vi "PTSequencer.check stop conditions.vi"(1 "conditions":T1[](array[typedef])) -> (0 "fulfilled":bool)   [LabVIEW 2014, in "PTSequencer.lvlib"]
uses:
  PTSequencer.lvlib
  PTSequencer.DIM service condition.ctl
  CSCore/CSSystem/CoreDefs/CoreDefs.rawDataType.ctl
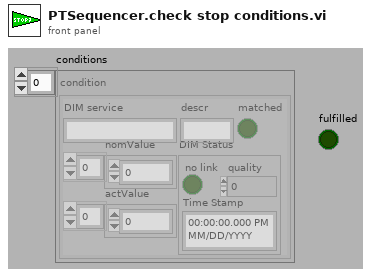
[diagram p1: front panel]
types:
  T1 = typedef "PTSequencer.lvlib/PTSequencer.DIM service condition.ctl" = cluster{"DIM service":string, "descr":string, "nomValue":T2, "actValue":T2, "matched":bool, "DIM Status":cluster{"no link":bool, "quality":i32, "Time Stamp":timestamp}}
  T2 = typedef "CoreDefs.rawDataType.ctl" = i8[]
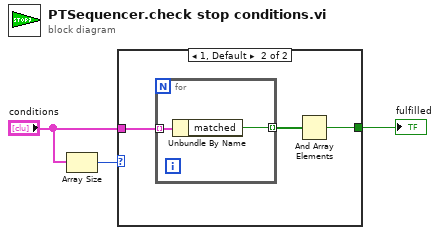
[diagram p0: block diagram]
diagram:
  n1 = Array Size(array="conditions") -> (size(s)=w1:i32)
  n2 = case shown="1, Default" w1 {
    tunnel: "conditions" -> [_ w6]
    tunnel: [_ w4] -> w3
    frame 0 {
    }
    frame 1, Default {
      n3 = for {
        tunnel: w6 -> [w8] mode=indexing
        tunnel: [w7] -> w5 mode=indexing
        n4 = Unbundle By Name(w8) -> ("matched"=w7:bool)
      }
      n5 = And Array Elements(Boolean array=w5) -> (logical AND=w4:bool)
    }
  }
  "fulfilled" <- w3
